vi "陀螺儀.vi"() -> ()   [LabVIEW 2018]
uses:
  <vilib>/myRIO/Express VI/Onboard IO/UART/UART Express VI.xnode
  <vilib>/ptbypt/NI_PtbyPt.lvlib
  <vilib>/myRIO/Instrument Drivers/Onboard IO/UART/typedef/VISA Configuration.ctl
  <vilib>/Instr/_visa.llb/VISA Configure Serial Port (Instr).vi
panel:
  in  "RESET":bool
  in  "plus":dbl
  in  "multiple":dbl
  out "¨¤«×(¬ü¤Æ¹L£x)":dbl
  out "±ÛÂà¨¤«×":dbl(knob) scale=-180.0..180.0
  out "¨¤«×":dbl
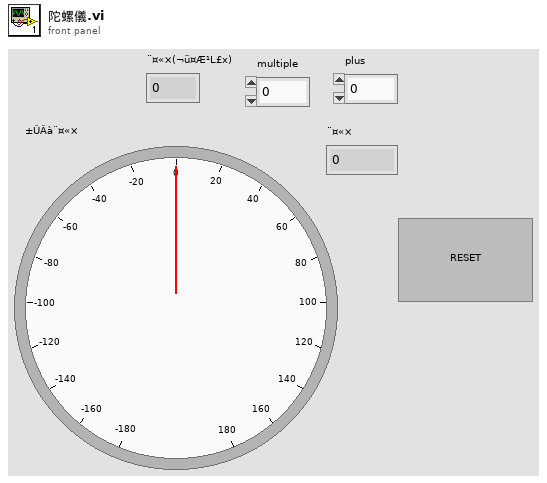
[diagram p1: front panel]
types:
  T1 = typedef "UART.lvlib/VISA Configuration.ctl" = cluster{"baud rate (9600)":u32, "data bits (8)":u16, "parity (0:none)":enum16{"None", "Odd", "Even", "Mark", "Space"}, "stop bits (10: 1 bit)":u16, "flow control (0:none)":u16, "termination char\n(0xA = '\\n' = LF) ":u8, "Enable Termination\nChar (T)":bool, "timeout (10sec)":u32}
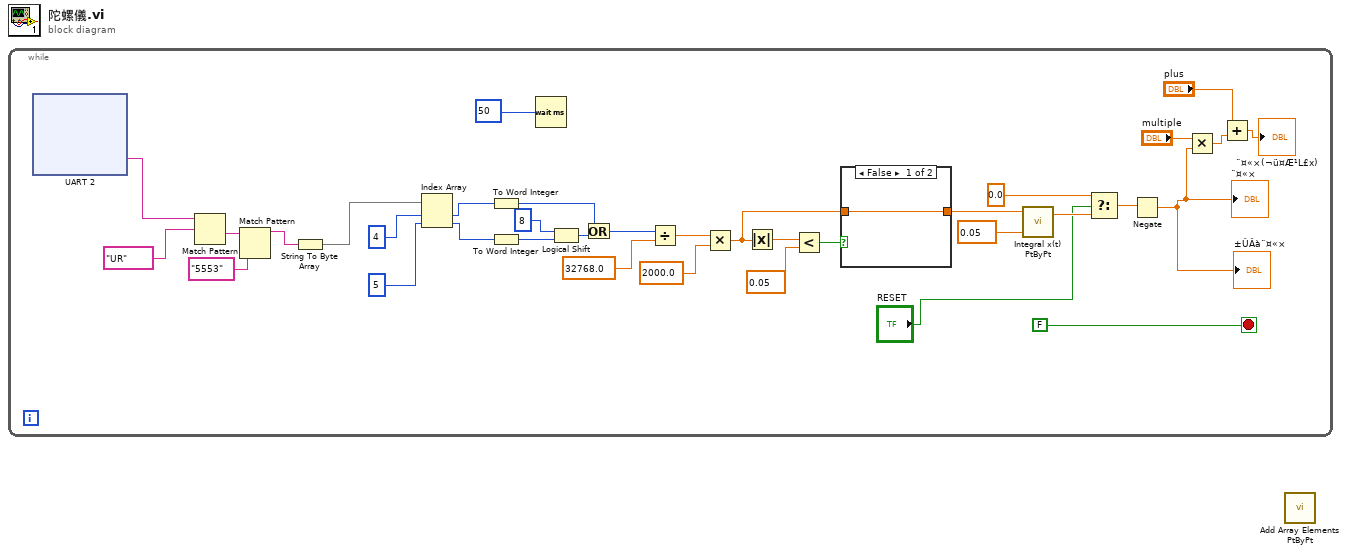
[diagram p0: block diagram]
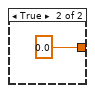
[diagram p2: hidden frame]
diagram:
  n1 = while {
    stop <- FALSE stop-if-true
    n2 = xnode "UART 2"() -> ("Characters Read"=w34:string)  [unwired: 1 in, 1 out]
    n3 = Match Pattern(string=w34, regular expression="UR") -> (after substring=w10:string)  [unwired: 1 in, 3 out]
    n4 = Match Pattern(string=w10, regular expression="5553") -> (before substring=w9:string)  [unwired: 1 in, 3 out]
    n5 = String To Byte Array(string=w9) -> (unsigned byte array=w14:u8[])
    n6 = Index Array(array=w14, index #1=4, index #2=5) -> (element #1=w31:u8, element #2=w12:u8)
    n7 = To Word Integer(number=w31) -> (16bit integer=w28:i16)
    n8 = To Word Integer(number=w12) -> (16bit integer=w30:i16)
    n9 = Wait (ms)(milliseconds to wait=u32 50) -> ()  [unwired: 1 out]
    n10 = Logical Shift(y=8, x=w30) -> (x << y=w27:i16)
    n11 = Or(x=w28, y=w27) -> (x .or. y?=w26:i16)
    n12 = Divide(x=w26, y=32768.0) -> (x/y=w24:dbl)
    n13 = Multiply(x=w24, y=2000.0) -> (x*y=w19:dbl)
    n14 = Absolute Value(x=w19) -> (abs(x)=w22:dbl)
    n15 = Less?(x=w22, y=0.05) -> (x < y?=w20:bool)
    n16 = case shown="False" w20 {
      tunnel: [w36 0.0] -> w18
      tunnel: w19 -> [w36 _]
      frame False {
      }
      frame True {
      }
    }
    n17 = call <vilib>:"Integral x(t) PtByPt.vi"("dt"=0.05, "x"=w18) -> ("integral x(t)"=w16:dbl)  [unwired: 2 in, 1 out]
    n18 = Select(t=0.0, s="RESET", f=w16) -> (s? t:f=w11:dbl)
    n19 = Negate(x=w11) -> (-x=w7:dbl)
    "¨¤«×" <- w7
    "±ÛÂà¨¤«×" <- w7
    n20 = Multiply(x="multiple", y=w7) -> (x*y=w5:dbl)
    n21 = Add(x="plus", y=w5) -> (x+y=→"¨¤«×(¬ü¤Æ¹L£x)":dbl)
  }
  n22 = call <vilib>:"Add Array Elements PtByPt.vi"() -> ()  [unwired: 4 in, 2 out]
